vi "Put.vi"(8 "error in (no error)":errorcluster, 10 "Data":variant, 11 "MsgPackSerializer in":refnum<class "MsgPackSerializer.lvclass">) -> (0 "error out":errorcluster, 3 "MsgPackSerializer out":refnum<class "MsgPackSerializer.lvclass">)   [LabVIEW 2015, in "MsgPackSerializer.lvclass"]
uses:
  MsgPackSerializer.lvclass
  <vilib>/Utility/Data Type/NI_Data Type.lvlib
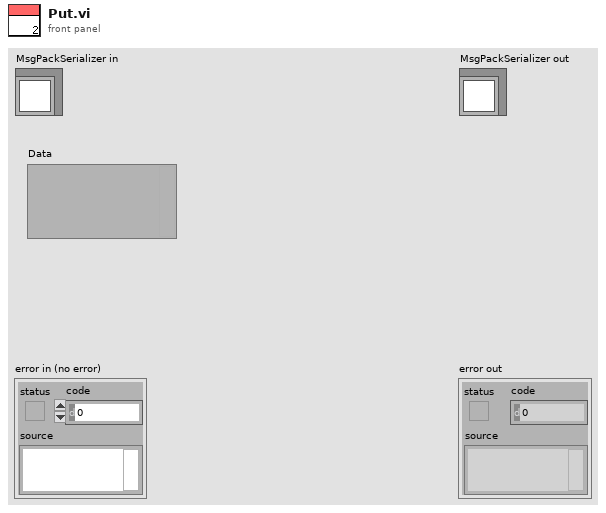
[diagram p1: front panel]
types:
  T1 = typedef "NI_Data Type.lvlib/Data Type.ctl" = enum8{"Invalid Type", "Void", "I8", "I16", "I32", "I64", "U8", "U16", "U32", "U64", "Single Float", "Double Float", "Extended Float", "Single Complex", "Double Complex", "Extended Complex", "Enum U8", "Enum U16", "Enum U32", "Enum U64", "Single Float With Unit", "Double Float With Unit", "Extended Float With Unit", "Single Complex with Unit", "Double Complex with Unit", "Extended Complex with Unit", "Boolean", "String", "Path", "Picture", "Tag", "Array", "Cluster", "Variant", "LV Variant", "Waveform", "Timestamp", "Digital Waveform", "Digital Data", "ExpressData", "Refnum", "External Data", "VI", "Poly VI", "LabVIEW Class Instance", "Fixed Point"}
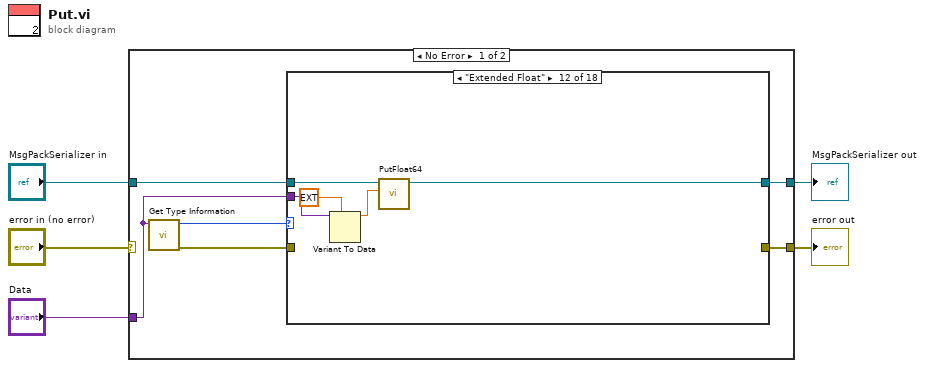
[diagram p0: block diagram]
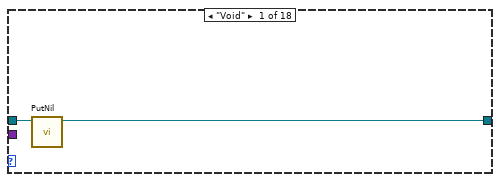
[diagram p2: hidden frame]
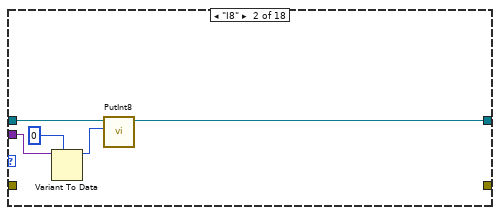
[diagram p3: hidden frame]
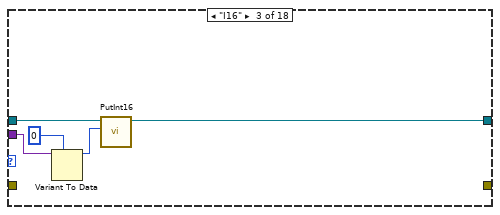
[diagram p4: hidden frame]
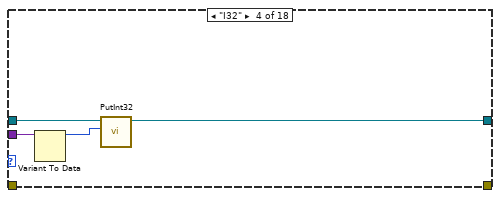
[diagram p5: hidden frame]
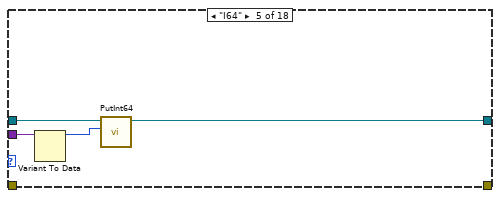
[diagram p6: hidden frame]
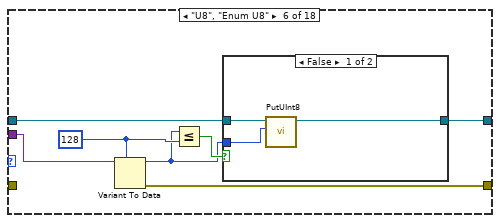
[diagram p7: hidden frame]
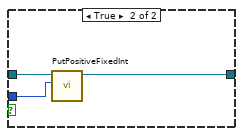
[diagram p8: hidden frame]
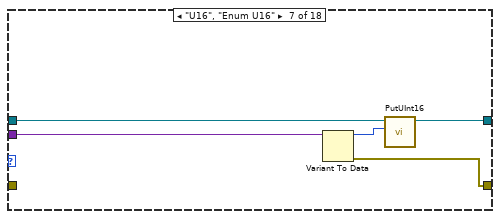
[diagram p9: hidden frame]
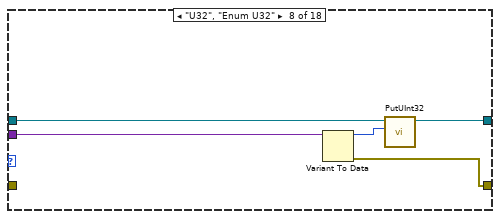
[diagram p10: hidden frame]
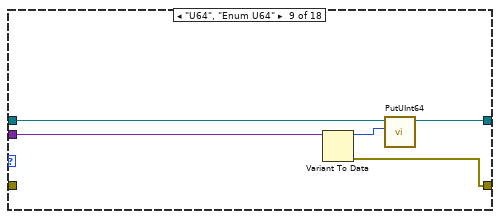
[diagram p11: hidden frame]
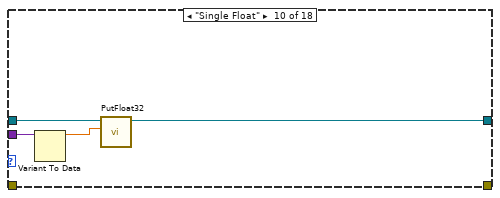
[diagram p12: hidden frame]
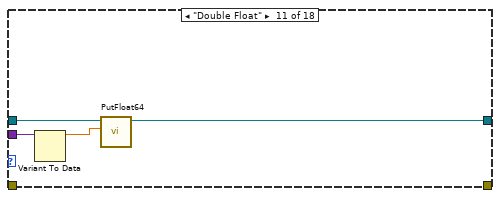
[diagram p13: hidden frame]
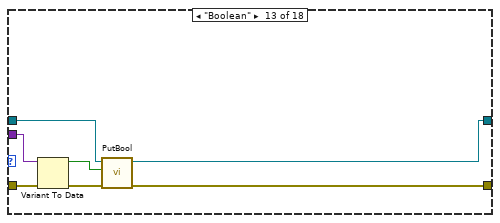
[diagram p14: hidden frame]
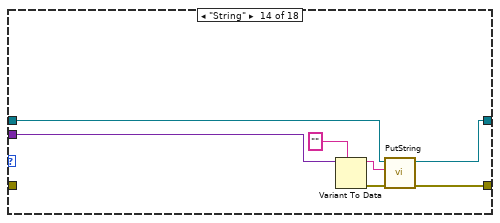
[diagram p15: hidden frame]
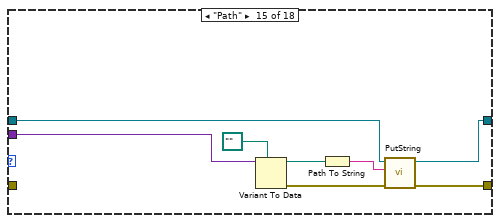
[diagram p16: hidden frame]
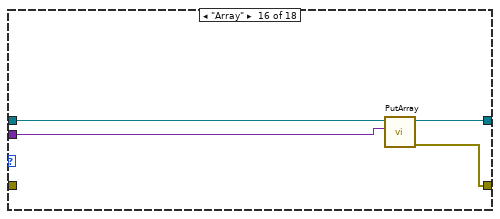
[diagram p17: hidden frame]
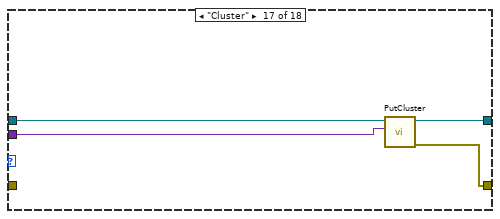
[diagram p18: hidden frame]
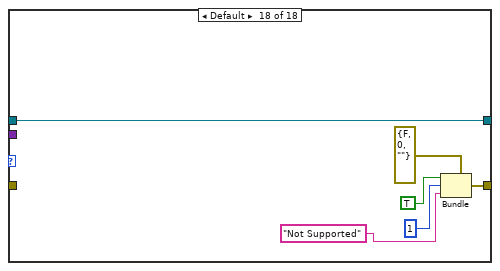
[diagram p19: hidden frame]
diagram:
  n1 = case shown="No Error" "error in (no error)" {
    selector: "error in (no error)" -> [_ w110]
    tunnel: [w7 w110] -> w4
    tunnel: [w9 w109] -> w2
    tunnel: "MsgPackSerializer in" -> [w10 w109]
    tunnel: "Data" -> [w8 _]
    frame No Error {
      n2 = call <vilib>:"Get Type Information.vi"("Variant"=w8) -> ("error out"=w6:errorcluster, "Type"=w11:T1)  [unwired: 6 in, 3 out]
      n3 = case shown="\"I16\"" w11 {
        tunnel: w10 -> [w13 w18 w23 w27 w29 w34 w49 w54 w59 w63 w67 w69 w79 w80 w90 w97 w101 w103]
        tunnel: [w12 w15 w22 w26 w28 w33 w46 w53 w56 w60 w66 w68 w76 w81 w88 w96 w100 w103] -> w9
        tunnel: w8 -> [_ w17 w19 w24 w31 w37 w48 w52 w58 w62 w65 w70 w78 w86 w89 w98 w102 _]
        tunnel: [_ _ _ _ _ w32 w45 w50 w55 _ _ _ w75 w82 w87 w95 w99 w104] -> w7
        tunnel: w6 -> [_ _ _ _ _ _ _ _ _ _ _ _ w74 _ _ _ _ _]
        frame "Void" {
          n4 = call "PutNil.vi"("MsgPackSerializer in"=w13) -> ("MsgPackSerializer out"=w12:refnum<class "MsgPackSerializer.lvclass">)  [unwired: 9 in, 1 out]
        }
        frame "I8" {
          n5 = Variant To Data(type=i8 0 ("Number"), Variant=w17) -> (data=w14:i8)  [unwired: 1 in, 1 out]
          n6 = call "PutInt8.vi"("Number"=w14, "MsgPackSerializer in"=w18) -> ("MsgPackSerializer out"=w15:refnum<class "MsgPackSerializer.lvclass">)  [unwired: 8 in, 1 out]
        }
        frame "I16" {
          n7 = Variant To Data(type=i16 0 ("Number"), Variant=w19) -> (data=w20:i16)  [unwired: 1 in, 1 out]
          n8 = call "PutInt16.vi"("Number"=w20, "MsgPackSerializer in"=w23) -> ("MsgPackSerializer out"=w22:refnum<class "MsgPackSerializer.lvclass">)  [unwired: 8 in, 1 out]
        }
        frame "I32" {
          n9 = Variant To Data(Variant=w24) -> (data=w25:i32)  [unwired: 2 in, 1 out]
          n10 = call "PutInt32.vi"("Number"=w25, "MsgPackSerializer in"=w27) -> ("MsgPackSerializer out"=w26:refnum<class "MsgPackSerializer.lvclass">)  [unwired: 8 in, 1 out]
        }
        frame "I64" {
          n11 = Variant To Data(Variant=w31) -> (data=w30:i64)  [unwired: 2 in, 1 out]
          n12 = call "PutInt64.vi"("Number"=w30, "MsgPackSerializer in"=w29) -> ("MsgPackSerializer out"=w28:refnum<class "MsgPackSerializer.lvclass">)  [unwired: 8 in, 1 out]
        }
        frame "U8", "Enum U8" {
          w36 = u8 128 ("Number")
          n13 = Variant To Data(type=w36, Variant=w37) -> (data=w35:u8, error out=w32:errorcluster)  [unwired: 1 in]
          n14 = Less Or Equal?(x=w35, y=w36) -> (x <= y?=w38:bool)
          n15 = case shown="False" w38 {
            tunnel: w35 -> [w41 w42]
            tunnel: w34 -> [w40 w44]
            tunnel: [w39 w43] -> w33
            frame False {
              n16 = call "PutUInt8.vi"("Number"=w41, "MsgPackSerializer in"=w40) -> ("MsgPackSerializer out"=w39:refnum<class "MsgPackSerializer.lvclass">)  [unwired: 8 in, 1 out]
            }
            frame True {
              n17 = call "PutPositiveFixedInt.vi"("Number"=w42, "MsgPackSerializer in"=w44) -> ("MsgPackSerializer out"=w43:refnum<class "MsgPackSerializer.lvclass">)  [unwired: 8 in, 1 out]
            }
          }
        }
        frame "U16", "Enum U16" {
          n18 = Variant To Data(Variant=w48) -> (data=w47:u16, error out=w45:errorcluster)  [unwired: 2 in]
          n19 = call "PutUInt16.vi"("Number"=w47, "MsgPackSerializer in"=w49) -> ("MsgPackSerializer out"=w46:refnum<class "MsgPackSerializer.lvclass">)  [unwired: 8 in, 1 out]
        }
        frame "U32", "Enum U32" {
          n20 = Variant To Data(Variant=w52) -> (data=w51:u32, error out=w50:errorcluster)  [unwired: 2 in]
          n21 = call "PutUInt32.vi"("Number"=w51, "MsgPackSerializer in"=w54) -> ("MsgPackSerializer out"=w53:refnum<class "MsgPackSerializer.lvclass">)  [unwired: 8 in, 1 out]
        }
        frame "U64", "Enum U64" {
          n22 = Variant To Data(Variant=w58) -> (data=w57:u64, error out=w55:errorcluster)  [unwired: 2 in]
          n23 = call "PutUInt64.vi"("Number"=w57, "MsgPackSerializer in"=w59) -> ("MsgPackSerializer out"=w56:refnum<class "MsgPackSerializer.lvclass">)  [unwired: 8 in, 1 out]
        }
        frame "Single Float" {
          n24 = Variant To Data(Variant=w62) -> (data=w61:sgl)  [unwired: 2 in, 1 out]
          n25 = call "PutFloat32.vi"("Number"=w61, "MsgPackSerializer in"=w63) -> ("MsgPackSerializer out"=w60:refnum<class "MsgPackSerializer.lvclass">)  [unwired: 8 in, 1 out]
        }
        frame "Double Float" {
          n26 = Variant To Data(Variant=w65) -> (data=w64:dbl)  [unwired: 2 in, 1 out]
          n27 = call "PutFloat64.vi"("Number"=w64, "MsgPackSerializer in"=w67) -> ("MsgPackSerializer out"=w66:refnum<class "MsgPackSerializer.lvclass">)  [unwired: 8 in, 1 out]
        }
        frame "Extended Float" {
          n28 = Variant To Data(type=ext 0.0 ("data"), Variant=w70) -> (data=w72:ext)  [unwired: 1 in, 1 out]
          n29 = call "PutFloat64.vi"("Number"=w72, "MsgPackSerializer in"=w69) -> ("MsgPackSerializer out"=w68:refnum<class "MsgPackSerializer.lvclass">)  [unwired: 8 in, 1 out]
        }
        frame "Boolean" {
          n30 = Variant To Data(error in=w74, Variant=w78) -> (data=w77:bool, error out=w73:errorcluster)  [unwired: 1 in]
          n31 = call "PutBool.vi"("error in (no error)"=w73, "Boolean"=w77, "MsgPackSerializer in"=w79) -> ("error out"=w75:errorcluster, "MsgPackSerializer out"=w76:refnum<class "MsgPackSerializer.lvclass">)  [unwired: 7 in]
        }
        frame "String" {
          n32 = Variant To Data(type="" ("string"), Variant=w86) -> (data=w84:string, error out=w83:errorcluster)  [unwired: 1 in]
          n33 = call "PutString.vi"("error in (no error)"=w83, "string"=w84, "MsgPackSerializer in"=w80) -> ("error out"=w82:errorcluster, "MsgPackSerializer out"=w81:refnum<class "MsgPackSerializer.lvclass">)  [unwired: 7 in]
        }
        frame "Path" {
          n34 = Variant To Data(type=path "" ("path"), Variant=w89) -> (data=w92:path, error out=w94:errorcluster)  [unwired: 1 in]
          n35 = Path To String(path=w92) -> (string=w91:string)
          n36 = call "PutString.vi"("error in (no error)"=w94, "string"=w91, "MsgPackSerializer in"=w90) -> ("error out"=w87:errorcluster, "MsgPackSerializer out"=w88:refnum<class "MsgPackSerializer.lvclass">)  [unwired: 7 in]
        }
        frame "Array" {
          n37 = call "PutArray.vi"("Array"=w98, "MsgPackSerializer in"=w97) -> ("error out"=w95:errorcluster, "MsgPackSerializer out"=w96:refnum<class "MsgPackSerializer.lvclass">)  [unwired: 8 in]
        }
        frame "Cluster" {
          n38 = call "PutCluster.vi"("Cluster"=w102, "MsgPackSerializer in"=w101) -> ("error out"=w99:errorcluster, "MsgPackSerializer out"=w100:refnum<class "MsgPackSerializer.lvclass">)  [unwired: 8 in]
        }
        frame Default {
          n39 = Bundle(cluster=errorcluster {"status"=FALSE, "code"=0, "source"=""} ("error IO"), "status"=TRUE, "code"=1 ("error code (no error:0)"), "source"="Not Supported" ("error source (\" \")")) -> (w104:errorcluster)
        }
      }
    }
    frame Error {
    }
  }
  "error out" <- w4
  "MsgPackSerializer out" <- w2
